vi "DB Insert Into, Array Input.vi"(5 "Data Types (strictly typed)":T2[](array[typedef]), 7 "Values":string[](array[string]), 8 "error in (no error)":errorcluster, 9 "Columns to Update":string[](array[string]), 10 "Data Table":string, 11 "connection reference in":T1) -> (0 "error out":errorcluster, 2 "SQL Command":string, 3 "connection reference out":T1)   [LabVIEW 2009]
uses:
  <vilib>/addons/database/Auxilliary.llb/DB Tools DataTypes.ctl
  <vilib>/addons/database/Connection.llb/Conn ObjectReference.ctl
  <vilib>/addons/database/Recordset.llb/Rec Destroy - Connection.vi
  <vilib>/addons/database/Connection.llb/Conn Execute.vi
  <vilib>/addons/database/NI_Database_API.lvlib
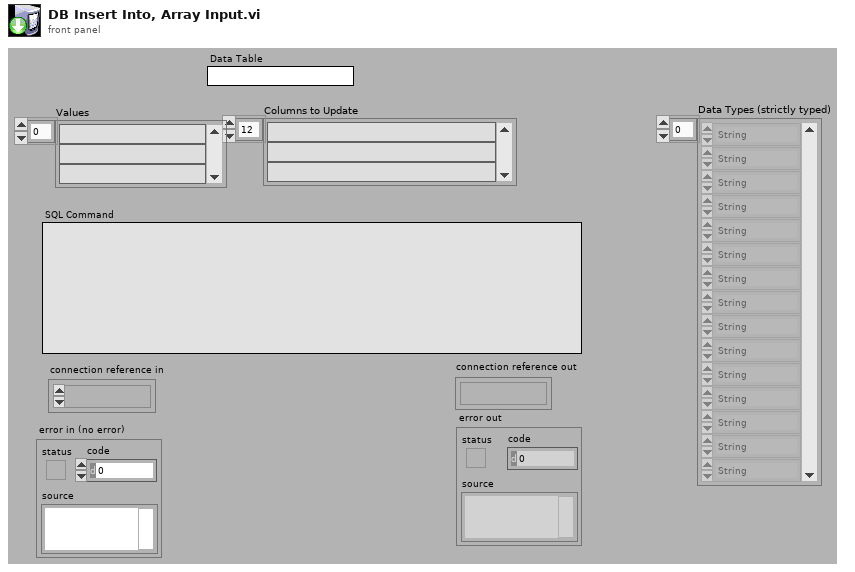
[diagram p1: front panel]
types:
  T1 = typedef "NI_Database_API.lvlib/Conn ObjectReference.ctl" = refnum<k1>
  T2 = typedef "NI_Database_API.lvlib/DB Tools DataTypes.ctl" = enum16{"String", "Long (I32)", "Single (SGL)", "Double (DBL)", "Date/Time", "Binary"}
  T3 = typedef "NI_Database_API.lvlib/Rec ObjectReference.ctl" = refnum<k1>
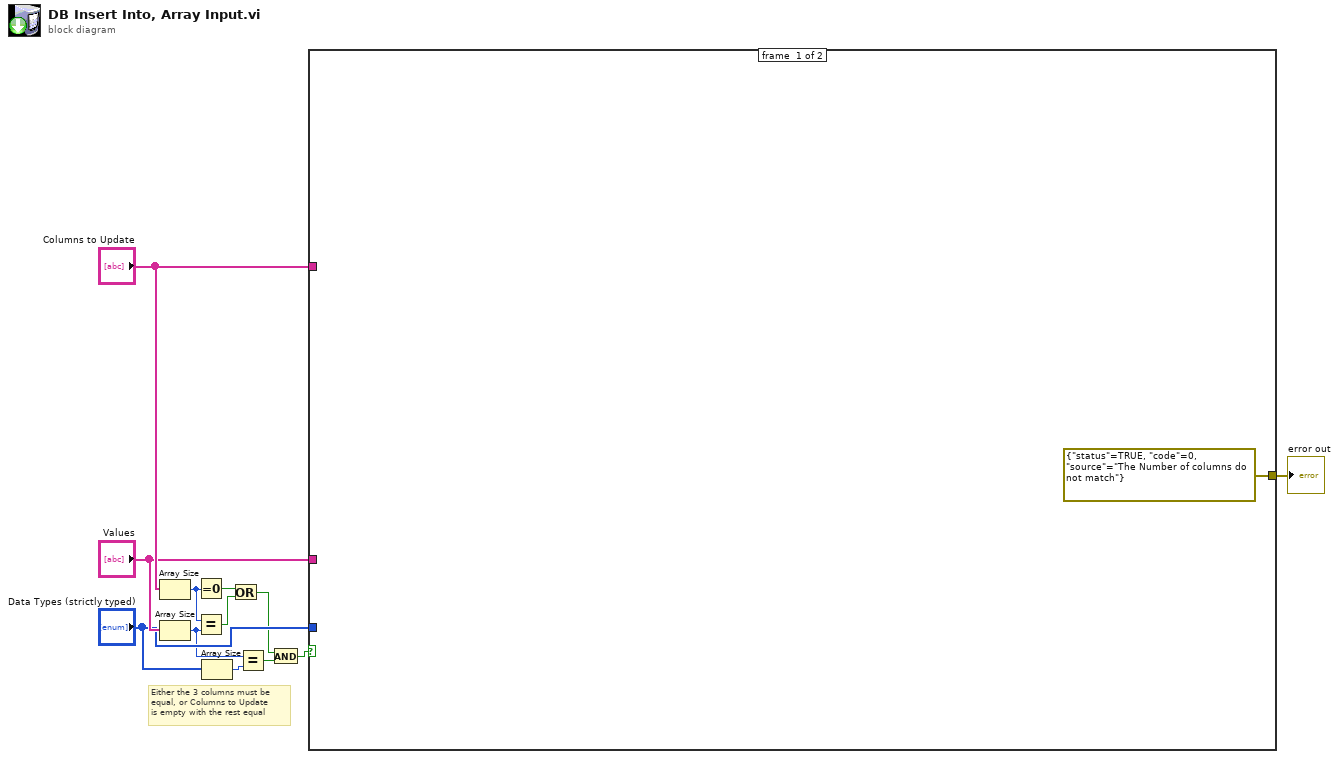
[diagram p0: block diagram]
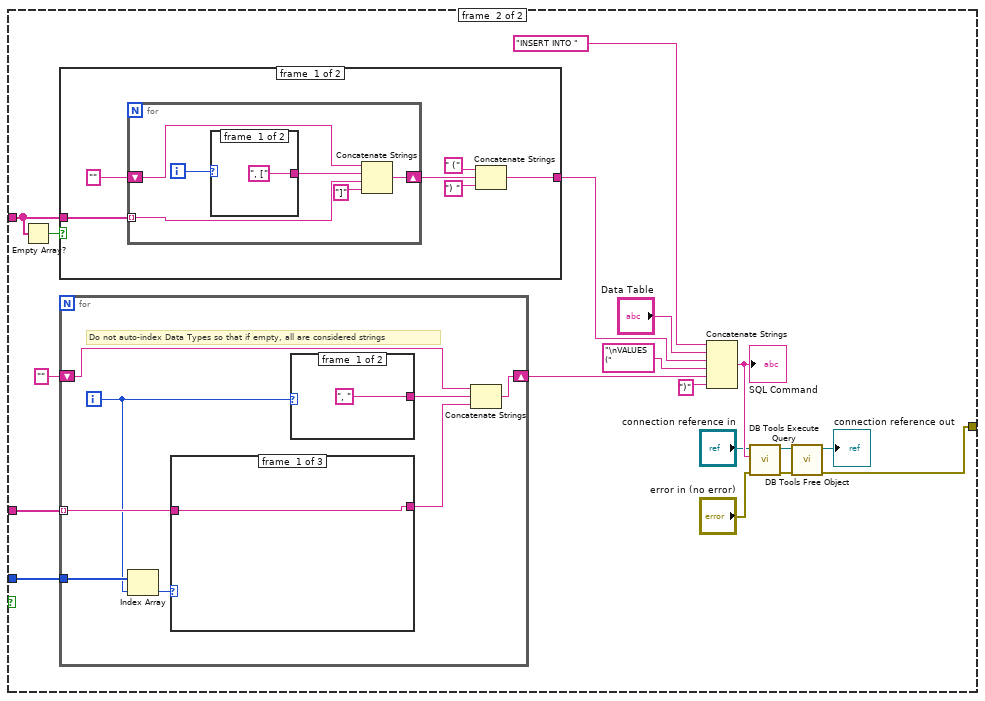
[diagram p2: hidden frame]
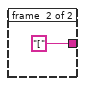
[diagram p3: hidden frame]
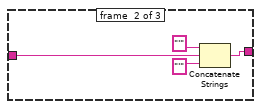
[diagram p5: hidden frame]
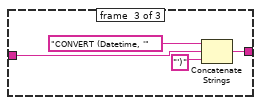
[diagram p6: hidden frame]
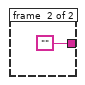
[diagram p7: hidden frame]
diagram:
  # "Either the 3 columns must be\nequal, or Columns to Update\nis empty with the rest equal"
  n1 = Array Size(array="Columns to Update") -> (size(s)=w1:i32)
  n2 = Array Size(array="Values") -> (size(s)=w8:i32)
  n3 = Equal To 0?(x=w1) -> (x = 0?=w4:bool)
  n4 = Equal?(x=w1, y=w8) -> (x = y?=w3:bool)
  n5 = Array Size(array="Data Types (strictly typed)") -> (size(s)=w9:i32)
  n6 = Or(x=w4, y=w3) -> (x .or. y?=w2:bool)
  n7 = Equal?(x=w8, y=w9) -> (x = y?=w7:bool)
  n8 = And(x=w2, y=w7) -> (x .and. y?=w6:bool)
  n9 = case shown="True" w6 {
    tunnel: "Columns to Update" -> [_ w17]
    tunnel: "Values" -> [_ w16]
    tunnel: "Data Types (strictly typed)" -> [_ w15]
    tunnel: [errorcluster {"status"=TRUE, "code"=0, "source"="The Number of columns do not match"} ("error out") w14] -> w5
    frame #0 {
    }
    frame #1 {
      n10 = Empty Array?(array=w17) -> (empty?=w25:bool)
      n11 = case shown="False" w25 {
        tunnel: w17 -> [w37 _]
        tunnel: [w33 _] -> w26
        frame #0 {
          n12 = for {
            tunnel: w37 -> [w43] mode=indexing
            shift-right: [w38] -> w35
            shift-left: "" -> [w39]
            i -> [w41]
            n13 = case shown="0" w41 {
              tunnel: [", [" ("string") "[" ("string")] -> w40
              frame #0 {
              }
              frame #1 {
              }
            }
            n14 = Concatenate Strings(w39, w40, w43, "]" ("string")) -> (w38:string)
          }
          n15 = Concatenate Strings(" (" ("string"), w35, ") " ("string")) -> (w33:string)
        }
        frame #1 {
        }
      }
      n16 = for {
        tunnel: w16 -> [w50] mode=indexing
        shift-right: [w51] -> w28
        shift-left: "" -> [w52]
        tunnel: w15 -> [w48]
        i -> [w46]
        # "Do not auto-index Data Types so that if empty, all are considered strings"
        n17 = Index Array(array=w48, index=w46) -> (element=w47:T2)
        n18 = case shown="\"Date/Time\"" w47 {
          tunnel: w50 -> [w54 w56 w60]
          tunnel: [w54 w55 w59] -> w49
          frame #0 {
          }
          frame #1 {
            n19 = Concatenate Strings("'" ("string"), w56, "'" ("string")) -> (w55:string)
          }
          frame #2 {
            n20 = Concatenate Strings("CONVERT (Datetime, '" ("string"), w60, "')" ("string")) -> (w59:string)
          }
        }
        n21 = case shown="Default" w46 {
          tunnel: [", " ("string") ""] -> w53
          frame #0 {
          }
          frame #1 {
          }
        }
        n22 = Concatenate Strings(w52, w53, w49) -> (w51:string)
      }
      n23 = Concatenate Strings("INSERT INTO ", "Data Table", w26, "\nVALUES (" ("string"), w28, ")" ("string")) -> (w22:string)
      "SQL Command" <- w22
      n24 = call-poly <vilib>:"DB Tools Execute Query.vi"("error in (no error)"="error in (no error)", "SQL query"=w22, "connection reference"="connection reference in") -> ("error out"=w19:errorcluster, "recordset reference"=w23:T3)  [unwired: 5 in]
      n25 = call-poly <vilib>:"DB Tools Free Object.vi"("error in (no error)"=w19, "recordset reference"=w23) -> ("error out"=w14:errorcluster, "connection reference"=→"connection reference out":T1)  [unwired: 8 in]
    }
  }
  "error out" <- w5
